vi "Add LabVIEW Error.vi"(8 "error in (no error)":errorcluster, 10 "LabVIEW Error":errorcluster, 11 "Alarm Handler Actor in":refnum<class "Alarm Handler Actor.lvclass">) -> (0 "error out":errorcluster, 3 "Alarm Handler Actor out":refnum<class "Alarm Handler Actor.lvclass">)   [LabVIEW 2015, in "Alarm Handler Actor.lvclass"]
uses:
  Alarm Handler Actor.lvclass
  Active Alarm.ctl
  Alarm Details.ctl
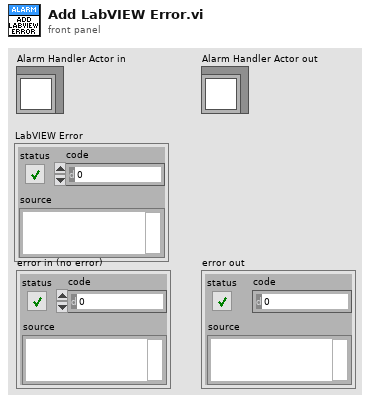
[diagram p1: front panel]
types:
  T1 = typedef "Alarm Handler Actor.lvclass/Active Alarm.ctl" = cluster{"Alarm Detail":T2, "Count":i32, "First Error":timestamp, "Last Error":timestamp, "LabVIEW Error":bool}
  T2 = typedef "Alarm Handler Actor.lvclass/Alarm Details.ctl" = cluster{"Code":i32, "Loop":i32, "Description":string, "Severity":i32, "Clear on Ack?":bool, "Log All Events?":bool}
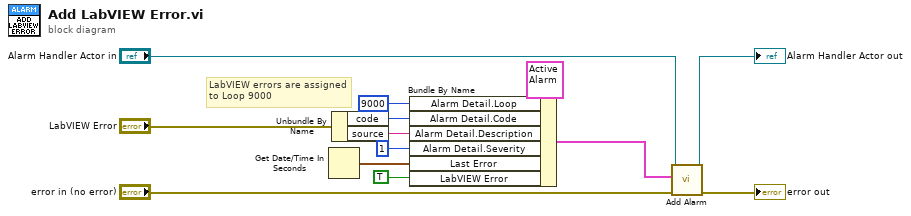
[diagram p0: block diagram]
diagram:
  # "LabVIEW errors are assigned to Loop 9000"
  n1 = Get Date/Time In Seconds() -> (seconds since 1Jan1904=w5:timestamp)
  n2 = Unbundle By Name("LabVIEW Error") -> ("code"=w4:i32, "source"=w8:string)
  n3 = Bundle By Name(cluster=T1 {"Alarm Detail"={"Code"=0, "Loop"=0, "Description"="", "Severity"=0, "Clear on Ack?"=FALSE, "Log All Events?"=FALSE}, "Count"=0, "First Error"=timestamp(0 s since 1904-01-01), "Last Error"=timestamp(0 s since 1904-01-01), "LabVIEW Error"=FALSE} ("Present Alarm"), "Alarm Detail.Loop"=9000 ("Error Detail.Loop"), "Alarm Detail.Code"=w4, "Alarm Detail.Description"=w8, "Alarm Detail.Severity"=1 ("Error Detail.Severity"), "Last Error"=w5, "LabVIEW Error"=TRUE ("LV error")) -> (w10:T1)
  n4 = call "Add Alarm.vi"("error in (no error)"="error in (no error)", "Alarm"=w10, "Actor in"="Alarm Handler Actor in") -> ("error out"=→"error out":errorcluster, "Actor out"=→"Alarm Handler Actor out":refnum<class "Alarm Handler Actor.lvclass">)  [unwired: 7 in]
